vi "average direction.vi"(2 "weight of each direction":dbl[](array[slide]) scale=0.0..10.0, 3 "directions":dbl[](array[knob]) scale=0.0..6.283) -> (0 "total weight":dbl, 1 "average direction":dbl(knob) scale=0.0..6.283)   [LabVIEW 2009]
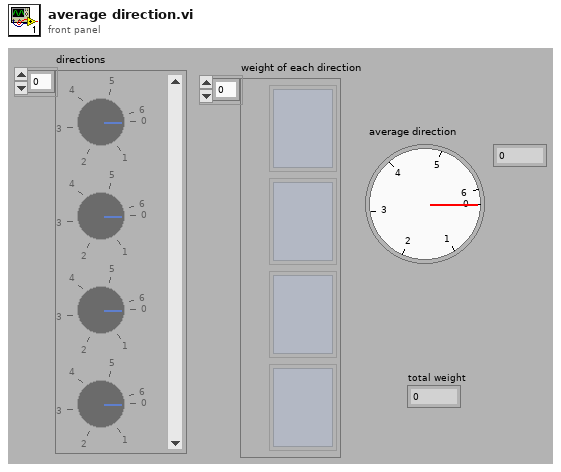
[diagram p1: front panel]
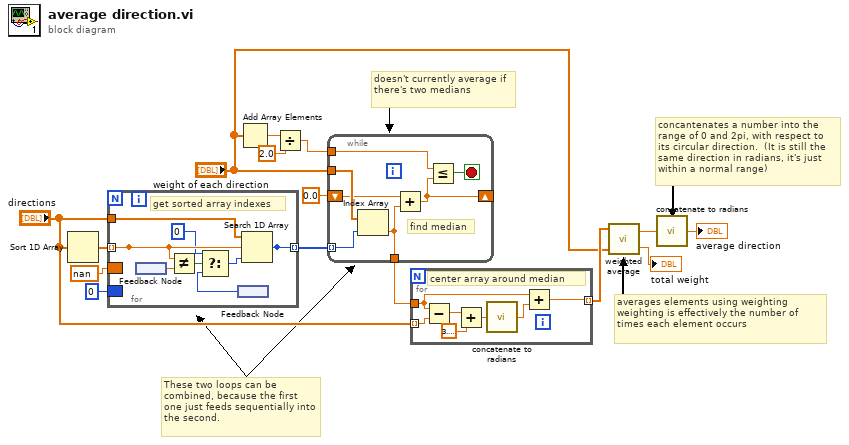
[diagram p0: block diagram]
diagram:
  # "doesn't currently average if there's two medians"
  # "These two loops can be combined, because the first one just feeds sequentially into the second."
  # "concantenates a number into the range of 0 and 2pi, with respect to its circular direction.  (It is still the same direction in radians, it's just within a normal range)"
  # "averages elements using weighting weighting is effectively the number of times each element occurs"
  n1 = Sort 1D Array(array="directions") -> (sorted array=w13:dbl[])
  n2 = for {
    tunnel: w13 -> [w21] mode=indexing
    tunnel: "directions" -> [w23]
    tunnel: [w20] -> w10 mode=indexing
    border: 0 ("index of element") -> [_]
    border: nan ("Numeric") -> [_]
    # "get sorted array indexes"
    n3 = feedback #1() -> (w22:dbl)
    n4 = Not Equal?(x=w21, y=w22) -> (x != y?=w17:bool)
    n5 = feedback #2() -> (w18:i32)
    n6 = Select(t=0, s=w17, f=w18) -> (s? t:f=w19:i32)
    n7 = Search 1D Array(1D array=w23, element=w21, start index (0)=w19) -> (index of element=w20:i32)
  }
  n8 = Add Array Elements(numeric array="weight of each direction") -> (sum=w12:dbl)
  n9 = Divide(x=w12, y=2.0) -> (x/y=w8:dbl)
  n10 = while {
    tunnel: "weight of each direction" -> [w30]
    tunnel: w10 -> [w28] mode=indexing
    shift-right: [w27] -> _
    shift-left: 0.0 ("y") -> [w29]
    tunnel: w8 -> [w25]
    tunnel: [w24] -> w6
    stop <- w26 stop-if-true
    # "find median"
    n11 = Index Array(array=w30, index=w28) -> (element=w24:dbl)
    n12 = Add(x=w29, y=w24) -> (x+y=w27:dbl)
    n13 = Less Or Equal?(x=w25, y=w27) -> (x <= y?=w26:bool)
  }
  n14 = for {
    tunnel: "directions" -> [w37] mode=indexing
    tunnel: w6 -> [w33]
    tunnel: [w32] -> w5 mode=indexing
    # "center array around median"
    n15 = Subtract(x=w33, y=w37) -> (x-y=w36:dbl)
    n16 = Add(x=w36, y=3.141592653589793) -> (x+y=w31:dbl)
    n17 = call "concatenate to radians.vi"("value"=w31) -> ("concatenated value"=w34:dbl)
    n18 = Add(x=w33, y=w34) -> (x+y=w32:dbl)
  }
  n19 = call "weighted average.vi"("weighting"="weight of each direction", "elements"=w5) -> ("total weight"=→"total weight":dbl, "average"=w15:dbl)  [unwired: 2 in]
  n20 = call "concatenate to radians.vi"("value"=w15) -> ("concatenated value"=→"average direction":dbl)
